vi "SIcamera_Driver.vi"(4 "error in (no error)":errorcluster, 6 "Action":enum16{"Launch", "Shutdown"}(ring)) -> (0 "error out":errorcluster, 2 "reference out (launch only)":refnum<vi>)   [LabVIEW 2015]
doc: "Provides an interface to the Grating Translation Manager. See the actions below.\n\nLaunch - launch the manager thread supplying references to the controls that the thread will update.\n\nHome - Home the grating translation stage\n\nMove - Move the grating to the position supplied by Grating#\n\nShutdown - Shutdown the grating translation manager"
uses:
  SystemUtil/Command.ctl
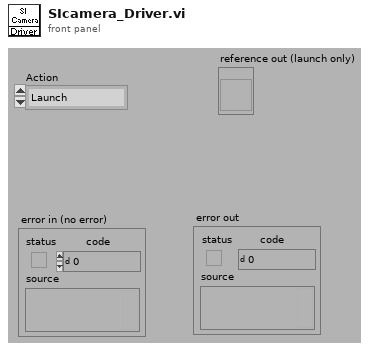
[diagram p1: front panel]
types:
  T1 = typedef "Command.ctl" = cluster{"Command":string, "Parameter":string}
  T2 = cluster{string, "type string":i16[], "data string":string}
  T3 = cluster{string, "type string":i16[], "data string":string}[]
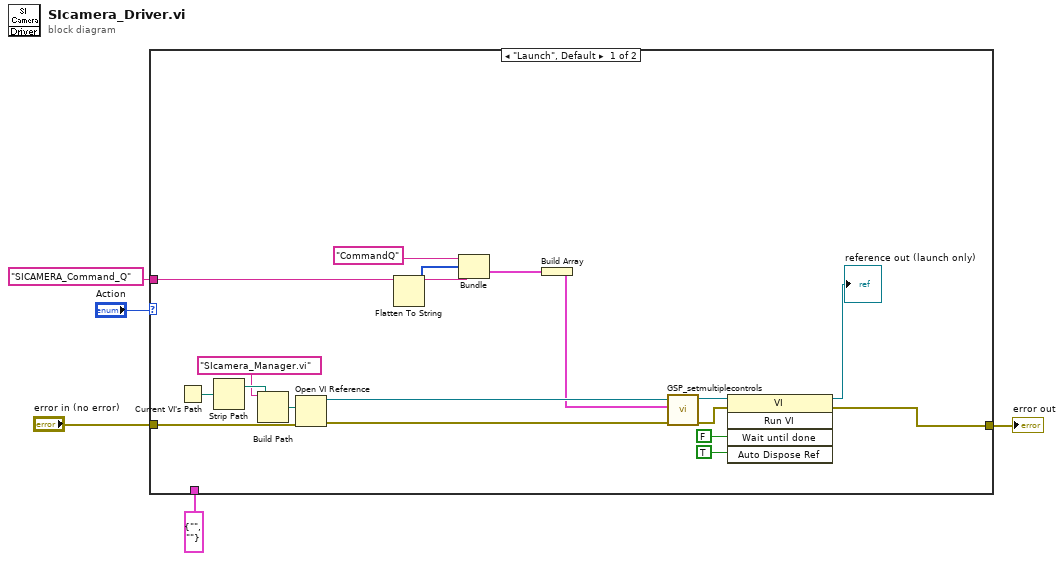
[diagram p0: block diagram]
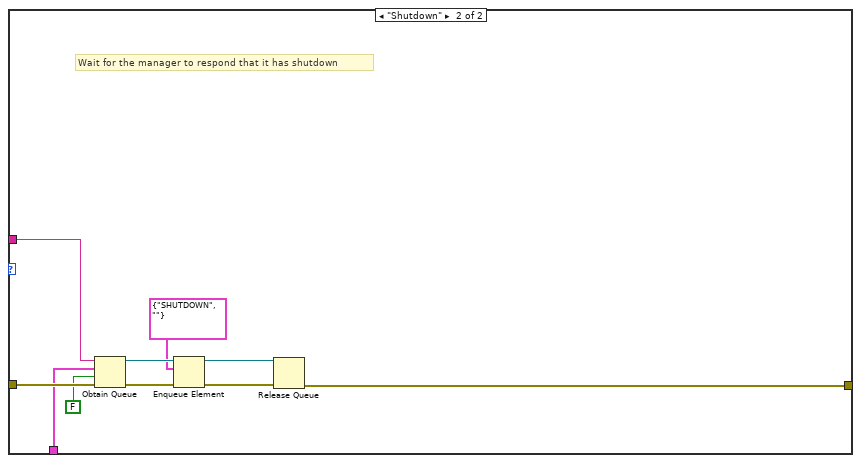
[diagram p2: hidden frame]
diagram:
  n1 = case shown="\"Launch\", Default" "Action" {
    tunnel: "error in (no error)" -> [w21 w34]
    tunnel: [w10 w25] -> w3
    tunnel: "SICAMERA_Command_Q" -> [w11 w31]
    tunnel: T1 {"Command"="", "Parameter"=""} ("Command") -> [_ w29]
    frame "Launch", Default {
      n2 = Current VI's Path() -> (path=w15:path)
      n3 = Strip Path(path=w15) -> (stripped path=w13:path)  [unwired: 1 out]
      n4 = Build Path(base path=w13, name or relative path="SIcamera_Manager.vi" ("vi path")) -> (appended path=w14:path)
      n5 = Open VI Reference(vi path=w14, error in (no error)=w21) -> (vi reference=w9:refnum<vi>, error out=w20:errorcluster)  [unwired: 4 in]
      n6 = Flatten To String(anything=w11) -> (data string=w22:string, type string=w23:i16[])  [unwired: 3 in, 1 out]
      n7 = Bundle("CommandQ", "type string"=w23, "data string"=w22) -> (w8:T2)  [unwired: 1 in]
      n8 = Build Array(w8) -> (w7:T3)
      n9 = call "GSP_setmultiplecontrols.vi"("error in (no error)"=w20, "Control Infos"=w7, "reference"=w9) -> ("error out"=w18:errorcluster, "reference out"=w19:refnum<vi>)  [unwired: 3 in]
      n10 = invoke class="VI" method="Run VI"(reference=w19, error in=w18, "Wait until done"=FALSE, "Auto Dispose Ref"=TRUE) -> (reference out=→"reference out (launch only)":refnum<vi>, error out=w10:errorcluster)  [unwired: 1 in, 3 out]
    }
    frame "Shutdown" {
      # "Wait for the manager to respond that it has shutdown"
      n11 = Obtain Queue(name (unnamed)=w31, element data type=w29, create if not found? (T)=FALSE, error in (no error)=w34) -> (queue out=w32:refnum<queue>, error out=w33:errorcluster)  [unwired: 1 in, 1 out]
      n12 = Enqueue Element(queue=w32, element=T1 {"Command"="SHUTDOWN", "Parameter"=""}, error in (no error)=w33) -> (queue out=w27:refnum<queue>, error out=w26:errorcluster)  [unwired: 1 in, 1 out]
      n13 = Release Queue(queue=w27, error in (no error)=w26) -> (error out=w25:errorcluster)  [unwired: 1 in, 2 out]
    }
  }
  "error out" <- w3
